vi "Write DAQmx_pulse_out.vi"(10 "DAQmx_pulse_out.lvclass":refnum<class "DAQmx_pulse_out.lvclass">, 11 "Experiment in":refnum<class "Experiment.lvclass">) -> (3 "Experiment out":refnum<class "Experiment.lvclass">)   [LabVIEW 2013, in "Experiment.lvclass"]
uses:
  Experiment.lvclass
  DAQmx_pulse_out/DAQmx_pulse_out.lvclass
  Experiment.lvclass/Experiment.ctl
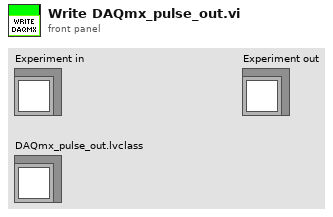
[diagram p1: front panel]
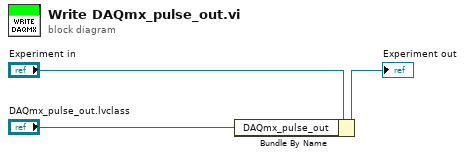
[diagram p0: block diagram]
diagram:
  n1 = Bundle By Name(cluster="Experiment in", "DAQmx_pulse_out"="DAQmx_pulse_out.lvclass") -> (→"Experiment out":refnum<class "Experiment.lvclass">)
